vi "Moving Ripple-Compute Max Level.vi"(0 "Moving Ripple":T3, 5 "Level in":T1) -> (4 "Max level":dbl, 6 "Level out":T1)   [LabVIEW 2020]
uses:
  Moving Ripple.ctl
  Moving Ripple.Params.ctl
  Moving Ripple.Data.ctl
  Controls/Level XCtl/Level Data.ctl
  Controls/Level XCtl/Level Units.ctl
  Utility VIs/Math VIs/Linear to dB (scalar).vi
  PXI DAQ VIs/DAQ Engine VIs/PXI Globals.vi
  Controls/Level XCtl/Level XCtl.xctl
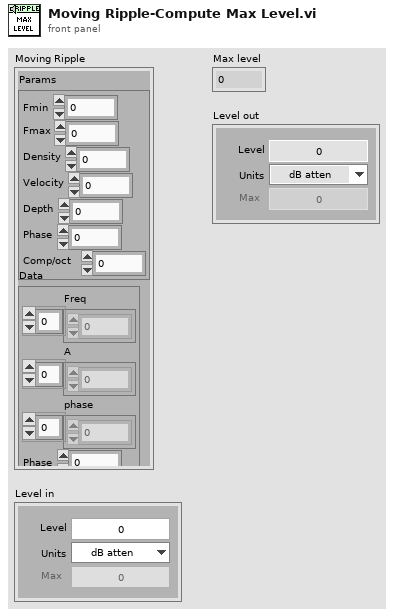
[diagram p1: front panel]
types:
  T1 = typedef "Level XCtl.xctl/Level Data.ctl" = cluster{"Level":dbl, "Units":T2, "Max":dbl, "Multiplier":dbl, "Cal File":path, "Cal":cluster{"Freq (Hz)":dbl[], "Mag (dB SPL)":dbl[], "Phase (deg)":dbl[]}}
  T2 = typedef "Level Units.ctl" = enum16{"dB atten", "dB SPL", "dB re 1 Vrms", "dB V/Hz½", "mW", "dB HL", "Volts", "dB mW"}
  T3 = typedef "Moving Ripple.ctl" = cluster{"Params":T4, "Data":T5}
  T4 = typedef "Moving Ripple.Params.ctl" = cluster{"Fmin":dbl, "Fmax":dbl, "Density":dbl, "Velocity":dbl, "Depth":dbl, "Phase":dbl, "Comp/oct":i32}
  T5 = typedef "Moving Ripple.Data.ctl" = cluster{"Freq":dbl[], "A":dbl[], "phase":dbl[], "Phase":dbl}
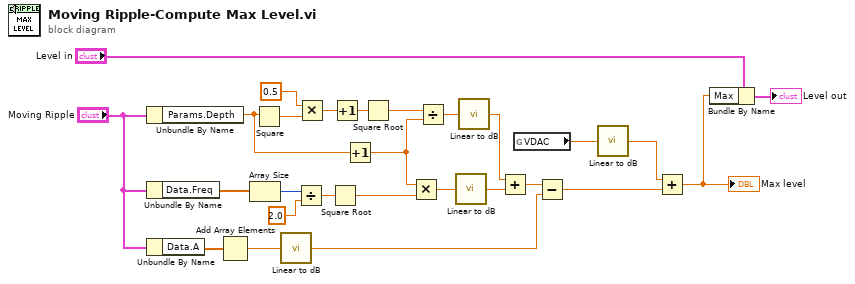
[diagram p0: block diagram]
diagram:
  n1 = Unbundle By Name("Moving Ripple") -> ("Params.Depth"=w22:dbl)
  n2 = Unbundle By Name("Moving Ripple") -> ("Data.Freq"=w20:dbl[])
  n3 = Unbundle By Name("Moving Ripple") -> ("Data.A"=w27:dbl[])
  n4 = Add Array Elements(numeric array=w27) -> (sum=w12:dbl)
  n5 = Array Size(array=w20) -> (size(s)=w19:i32)
  n6 = Square(x=w22) -> (x^2=w26:dbl)
  n7 = call-poly "Linear to dB.vi"("Linear"=w12) -> ("dB"=w11:dbl)
  n8 = Divide(x=w19, y=2.0) -> (x/y=w17:dbl)
  n9 = Multiply(x=0.5, y=w26) -> (x*y=w24:dbl)
  n10 = Square Root(x=w17) -> (sqrt(x)=w2:dbl)
  n11 = Increment(x=w24) -> (x+1=w23:dbl)
  n12 = Increment(x=w22) -> (x+1=w16:dbl)
  n13 = Square Root(x=w23) -> (sqrt(x)=w4:dbl)
  n14 = Multiply(x=w16, y=w2) -> (x*y=w15:dbl)
  n15 = Divide(x=w4, y=w16) -> (x/y=w14:dbl)
  n16 = call-poly "Linear to dB.vi"("Linear"=w15) -> ("dB"=w1:dbl)
  n17 = call-poly "Linear to dB.vi"("Linear"=w14) -> ("dB"=w3:dbl)
  n18 = Add(x=w3, y=w1) -> (x+y=w13:dbl)
  n19 = global read "PXI Globals.vi" "VDAC"() -> (w10:dbl)
  n20 = Subtract(x=w13, y=w11) -> (x-y=w8:dbl)
  n21 = call-poly "Linear to dB.vi"("Linear"=w10) -> ("dB"=w9:dbl)
  n22 = Add(x=w9, y=w8) -> (x+y=w6:dbl)
  "Max level" <- w6
  n23 = Bundle By Name(cluster="Level in", "Max"=w6) -> (→"Level out":T1)
